vi "BPSK_abhijit.vi"() -> ()   [LabVIEW 2012]
panel:
  in  "carrier":dbl(slide) scale=0.0..5000.0
  in  "binary data":dbl(slide) scale=0.0..500.0
  out "Demodulated":dynamicdata(graph)
  out "Binary data":dynamicdata(graph)
  out "Waveform Graph 3":dynamicdata(graph)
  out "BPSK":dynamicdata(graph)
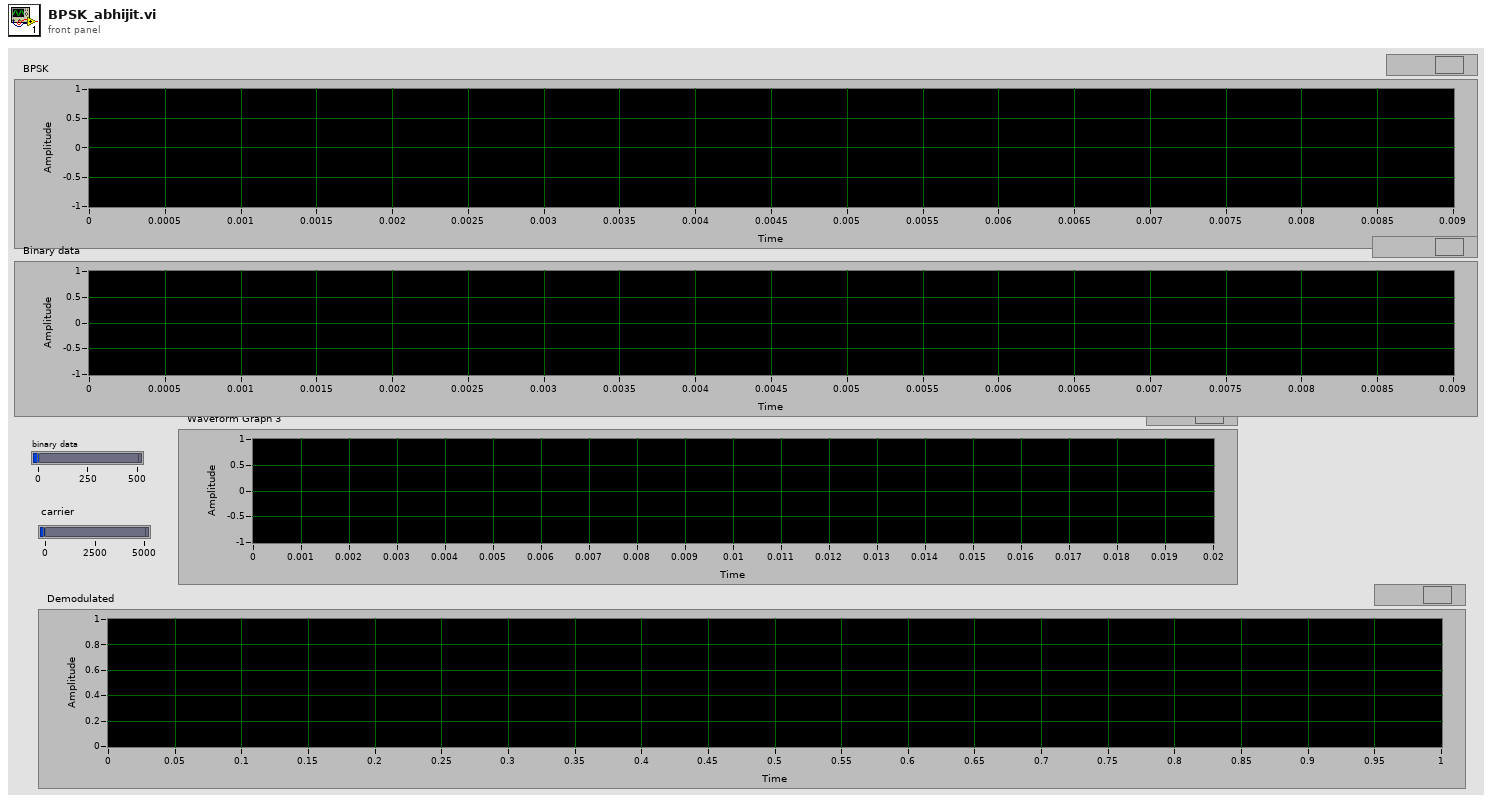
[diagram p1: front panel]
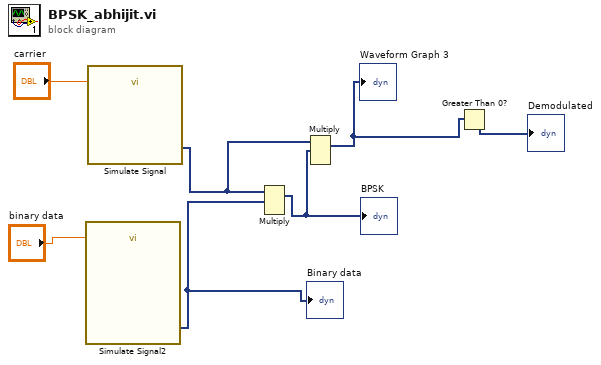
[diagram p0: block diagram]
diagram:
  n1 = call "Simulate Signal2"("Frequency"="binary data") -> ("Square"=w4:dynamicdata)  [unwired: 13 in, 1 out]
  "Binary data" <- w4
  n2 = call "Simulate Signal"("Frequency"="carrier") -> ("Sine"=w7:dynamicdata)  [unwired: 13 in, 1 out]
  n3 = Multiply(1:w4, 2:w7) -> (0:w6:dynamicdata)  [unwired: 1 in, 1 out]
  "BPSK" <- w6
  n4 = Multiply(1:w6, 2:w7) -> (0:w5:dynamicdata)  [unwired: 1 in, 1 out]
  "Waveform Graph 3" <- w5
  n5 = Greater Than 0?(x=w5) -> (x > 0?=→"Demodulated":dynamicdata)
